vi "Close.vi"(8 "Error In":errorcluster, 11 "object in":refnum<class "Scope Base.lvclass">) -> (0 "Error Out":errorcluster, 3 "object out":refnum<class "Scope Base.lvclass">)   [LabVIEW 2023, in "Scope Base.lvlib" / "Scope Base.lvclass"]
uses:
  Scope Base.lvclass
  Scope Base.lvclass/Scope Base.ctl
  Interfaces/IConfigure Scope/IConfigure Scope.lvclass
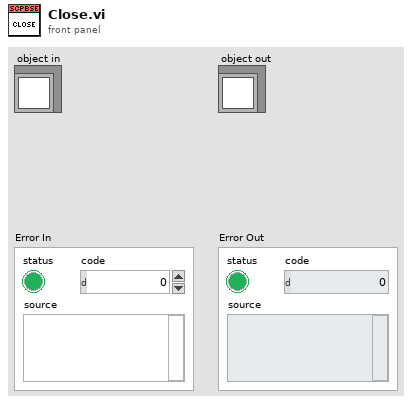
[diagram p1: front panel]
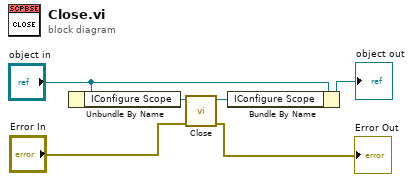
[diagram p0: block diagram]
diagram:
  n1 = Unbundle By Name("object in") -> ("IConfigure Scope"=w5:refnum<class "IConfigure Scope.lvclass">)
  n2 = call-dynamic "Close.vi"("error in (no error)"="Error In", "IConfigure in"=w5) -> ("error out"=→"Error Out":errorcluster, "IConfigure out"=w1:refnum<class "IConfigure Scope.lvclass">)  [unwired: 8 in]
  n3 = Bundle By Name(cluster="object in", "IConfigure Scope"=w1) -> (→"object out":refnum<class "Scope Base.lvclass">)
